vi "DB - [Config].[Parameter].vi"(5 "Application":string, 6 "[PlantId]":string, 7 "DB Connection":T2={"Open"=TRUE, "Close"=TRUE}, 8 "error in (no error)":errorcluster, 10 "[ParameterId] Values":string[](array[string])=["AllowWpsEdit", "DateFormat"], 11 "connection reference":T1) -> (0 "SUMMARY":errorcluster, 2 "2D data":string[][](array[string]), 3 "connection reference":T1)   [LabVIEW 2013]
doc: "----------------------------------\n-- Reinehold Systems Solutions\n-- 2015-01-13\n----------------------------------\nUSE [SRTRS]\nSELECT [ParameterId], [Value]\nFROM [Config].[Parameter]\nWHERE [PlantId] = '' AND\n[Inactive] = '0' AND\n[ParameterId] IN ('AllowWpsEdit' ,'DateFormat' )"
uses:
  <vilib>/addons/database/Connection.llb/Conn ObjectReference.ctl
  Controls/DB - OpenClose.ctl
  Controls/Global SRTRS.vi
  Controls/Global CMS.vi
  Controls/Global AMS.vi
  <vilib>/addons/database/Connection.llb/Conn Execute.vi
  <vilib>/addons/database/Recordset.llb/Rec Fetch Recordset Data (R).vi
  <vilib>/addons/database/Recordset.llb/Rec Destroy - Connection.vi
  <vilib>/addons/database/Connection.llb/DB Tools Open Connec (String).vi
  <vilib>/addons/database/_DB Variant To Data/Database Variant To Data.xnode
  <vilib>/addons/database/NI_Database_API.lvlib
panel:
  out "Close":errorcluster
  out "SQL Statement":string
  out "DB.Schema.Table\nDB.Config.Parameter":string="SRTRS.Config.Parameter"
  out "Connection Information":T3={"Connection "="SQL Server 32bit HPEnvy", "Username"="admin", "Password"="admin123"}
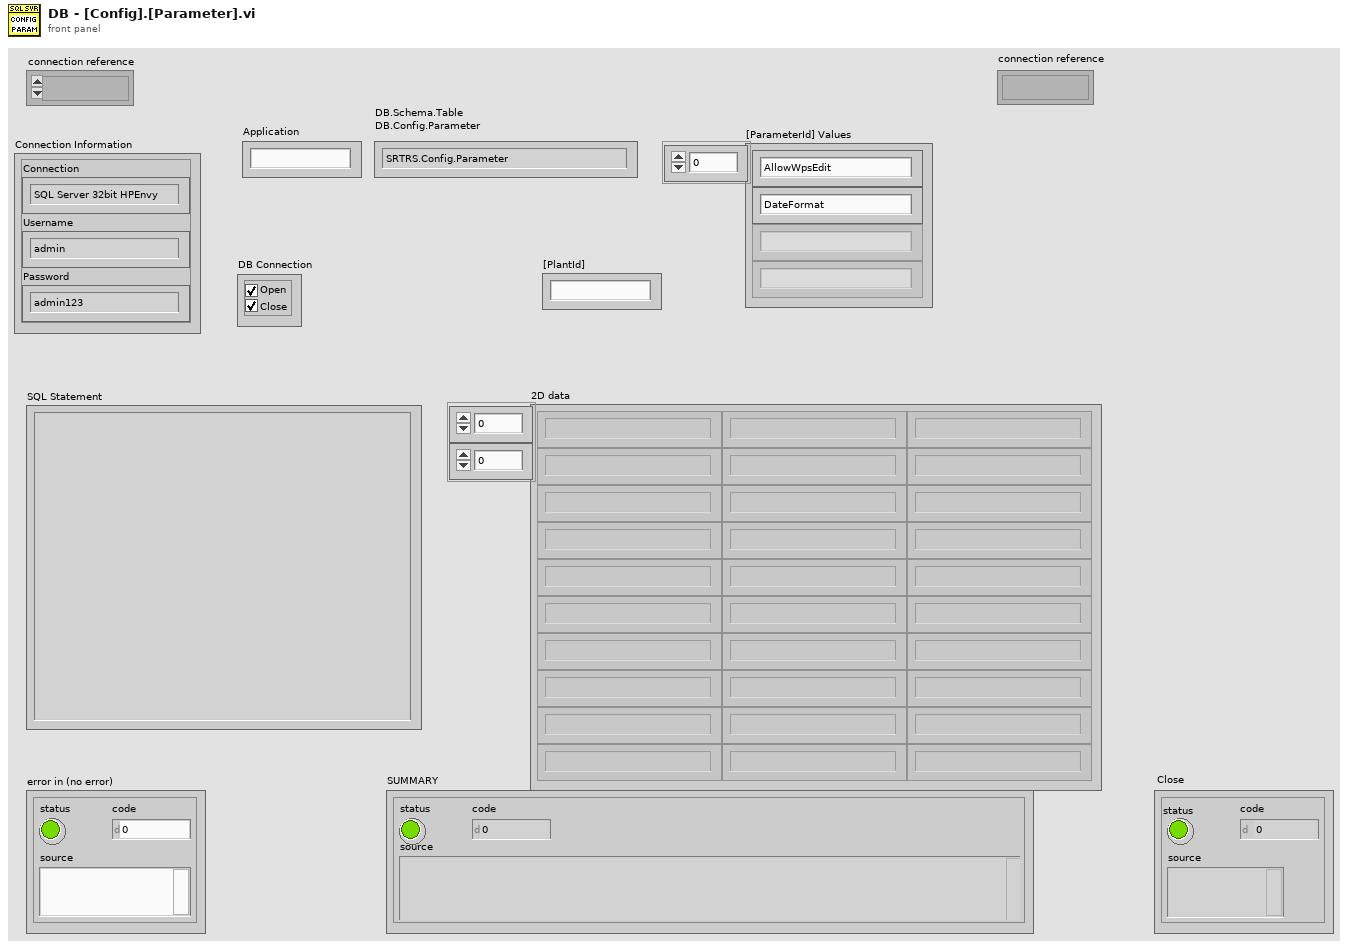
[diagram p1: front panel]
types:
  T1 = typedef "NI_Database_API.lvlib/Conn ObjectReference.ctl" = refnum<k1>
  T2 = typedef "DB - OpenClose.ctl" = cluster{"Open":bool, "Close":bool}
  T3 = cluster{"Connection ":string, "Username":string, "Password":string}
  T4 = typedef "Enum - InteractiveMode-SubVIMode.ctl" = enum16{"Interactive", "subVI Mode"}
  T5 = typedef "Connection Information Cluster.ctl" = cluster{"Connection ":string, "Username":string, "Password":string}
  T6 = typedef "DB - DB.Schema.Table.ctl" = cluster{"DB":string, "Schema":string, "Table":string}
  T7 = typedef "NI_Database_API.lvlib/Rec ObjectReference.ctl" = refnum<k1>
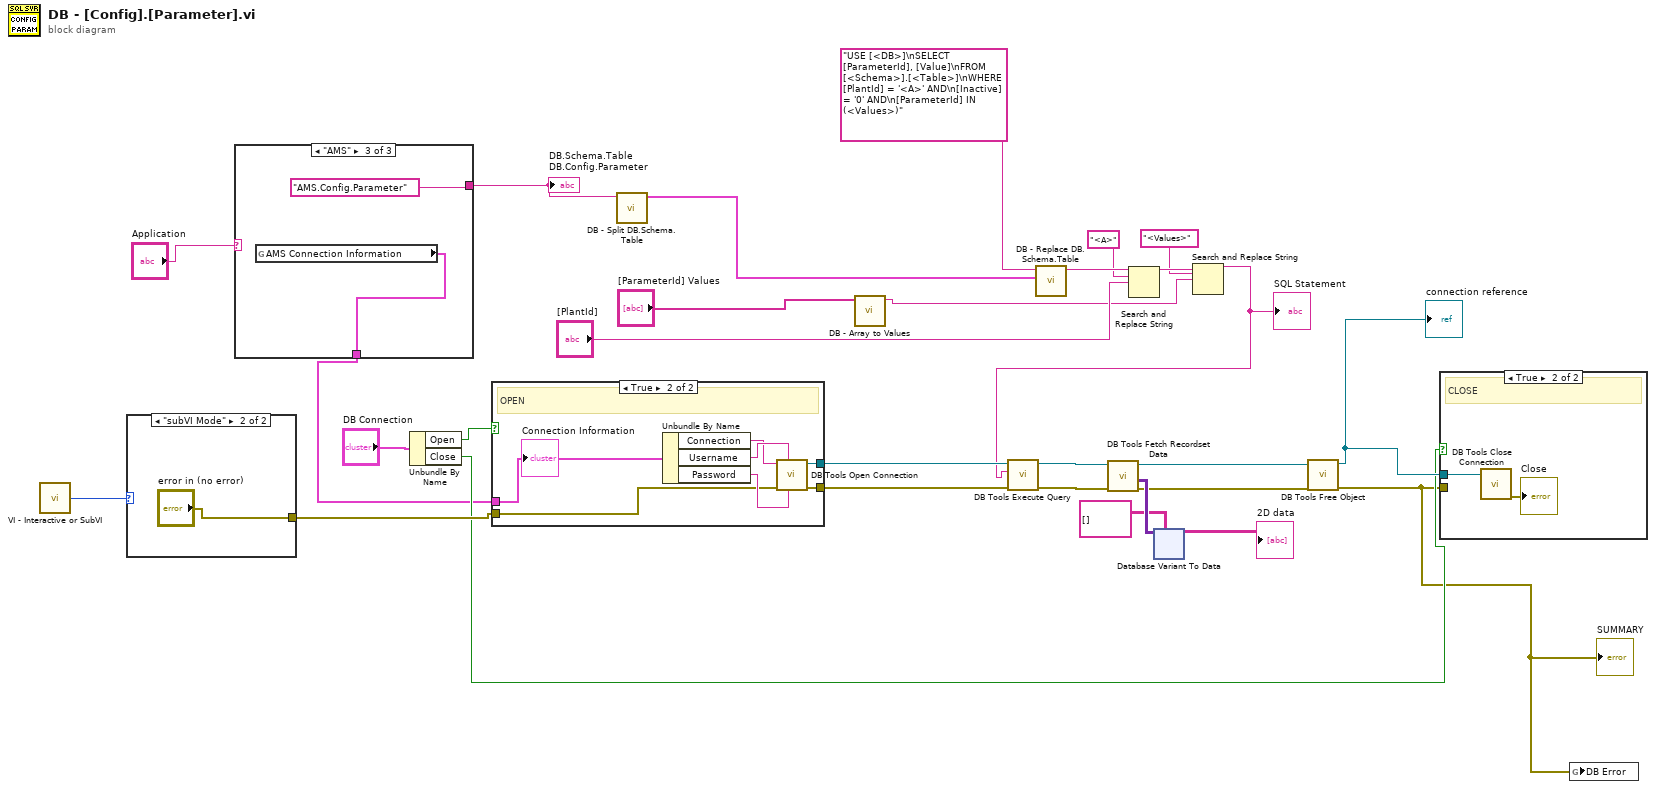
[diagram p0: block diagram]
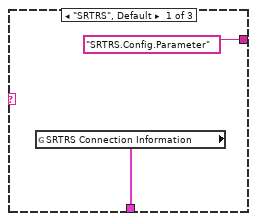
[diagram p2: hidden frame]
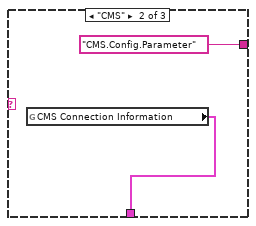
[diagram p3: hidden frame]
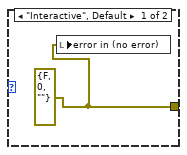
[diagram p5: hidden frame]
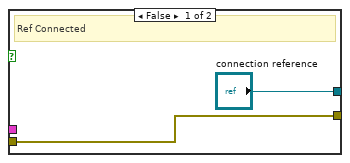
[diagram p6: hidden frame]
diagram:
  n1 = call "VI - Interactive or SubVI.vi"() -> ("Mode"=w27:T4)  [unwired: 5 in]
  n2 = case shown="\"subVI Mode\"" w27 {
    tunnel: [w30 "error in (no error)"] -> w26
    frame "Interactive", Default {
      w30 = errorcluster {"status"=FALSE, "code"=0, "source"=""} ("error in (no error)")
      n3 = local write "error in (no error)"(w30) -> ()
    }
    frame "subVI Mode" {
    }
  }
  n4 = case shown="\"AMS\"" "Application" {
    tunnel: ["SRTRS.Config.Parameter" ("DB.Schema.Table\nSRTRS.Config.Parameter") "CMS.Config.Parameter" ("DB.Schema.Table\nSRTRS.Config.Parameter") "AMS.Config.Parameter" ("DB.Schema.Table\nSRTRS.Config.Parameter")] -> w7
    tunnel: [w32 w34 w36] -> w6
    frame "SRTRS", Default {
      n5 = global read "Global SRTRS.vi" "SRTRS Connection Information"() -> (w32:T5)
    }
    frame "CMS" {
      n6 = global read "Global CMS.vi" "CMS Connection Information"() -> (w34:T5)
    }
    frame "AMS" {
      n7 = global read "Global AMS.vi" "AMS Connection Information"() -> (w36:T5)
    }
  }
  "DB.Schema.Table\nDB.Config.Parameter" <- w7
  n8 = Unbundle By Name("DB Connection") -> ("Open"=w28:bool, "Close"=w16:bool)
  n9 = case shown="True" w28 {
    tunnel: ["connection reference" w43] -> w19
    tunnel: w26 -> [w38 w42]
    tunnel: [w38 w41] -> w18
    tunnel: w6 -> [_ w40]
    frame False {
      # "Ref Connected"
    }
    frame True {
      # "OPEN"
      n10 = Unbundle By Name(w40) -> ("Connection"=w45:string, "Username"=w46:string, "Password"=w44:string)
      n11 = call-poly <vilib>:"DB Tools Open Connection.vi"("password"=w44, "userID"=w46, "error in (no error)"=w42, "connection information"=w45) -> ("error out"=w41:errorcluster, "connection reference"=w43:T1)  [unwired: 4 in]
      "Connection Information" <- w40
    }
  }
  n12 = call "DB - Split DB.Schema.Table.vi"("DB.Schema.Table"=w7) -> ("DB.Schema.Table"=w15:T6)  [unwired: 10 in]
  n13 = call "DB - Array to Values.vi"("Array (0xFFFE autodetect)"="[ParameterId] Values") -> ("<Values>"=w1:string)  [unwired: 10 in]
  n14 = call "DB - Replace DB.Schema.Table.vi"("DB.Schema.Table"=w15, "string in"="USE [<DB>]\nSELECT [ParameterId], [Value]\nFROM [<Schema>].[<Table>]\nWHERE [PlantId] = '<A>' AND\n[Inactive] = '0' AND\n[ParameterId] IN (<Values>)") -> ("string out"=w13:string)  [unwired: 8 in, 1 out]
  n15 = Search and Replace String(input string=w13, search string="<A>", replace string="[PlantId]") -> (result string=w3:string)  [unwired: 5 in, 3 out]
  n16 = Search and Replace String(input string=w3, search string="<Values>", replace string=w1) -> (result string=w4:string)  [unwired: 5 in, 3 out]
  "SQL Statement" <- w4
  n17 = call-poly <vilib>:"DB Tools Execute Query.vi"("error in (no error)"=w18, "SQL query"=w4, "connection reference"=w19) -> ("error out"=w25:errorcluster, "recordset reference"=w24:T7)  [unwired: 5 in]
  n18 = call-poly <vilib>:"DB Tools Fetch Recordset Data.vi"("error in (no error)"=w25, "recordset reference"=w24) -> ("error out"=w20:errorcluster, "recordset data"=w23:variant[][], "recordset reference out"=w21:T7)  [unwired: 3 in]
  n19 = xnode "Database Variant To Data"("database variant"=w23, "type"=string[][] []) -> ("data"=→"2D data":string[][])  [unwired: 1 in, 1 out]
  n20 = call-poly <vilib>:"DB Tools Free Object.vi"("error in (no error)"=w20, "recordset reference"=w21) -> ("error out"=w9:errorcluster, "connection reference"=w17:T1)  [unwired: 8 in]
  "SUMMARY" <- w9
  "connection reference" <- w17
  n21 = case shown="True" w16 {
    tunnel: w17 -> [_ w48]
    tunnel: w9 -> [_ _]
    frame False {
      # "Ref Connected"
    }
    frame True {
      # "CLOSE"
      n22 = call <vilib>:"DB Tools Close Connection.vi"("connection reference"=w48) -> ("error out"=→"Close":errorcluster)  [unwired: 6 in]
    }
  }
  n23 = global write "Global SRTRS.vi" "DB Error"(w9) -> ()
